vi "TSM SSC Digital Configure Single Level.vi"(0 "Digital TSM In":T2, 5 "Level Type to Set":T1, 7 "Setting":dbl, 11 "error in":errorcluster) -> (4 "Digital TSM Out":T2, 15 "error out":errorcluster)   [LabVIEW 2020]
doc: "Configures and applies the specified single level to the specified pin(s) and pin group(s)."
uses:
  TSM/TSM SSC Digital.ctl
  <vilib>/NI_TestStand_SemiconductorModule/NI_TestStand_Semiconductor_Module.lvlibp/PinMap/Digital Pattern/PinQueryContext/DigitalPatternPinQueryContext.lvclass
  SSC Digital/SSC Digital.ctl
  SSC Digital/Pin Levels and Timing/SSC Digital Single Level Selection.ctl
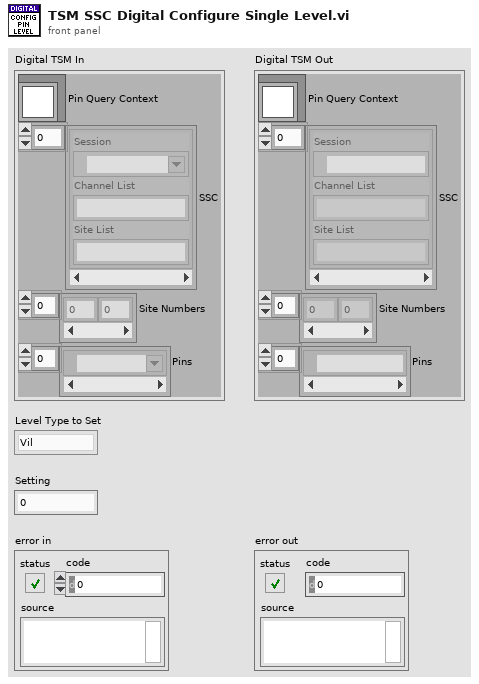
[diagram p1: front panel]
types:
  T1 = typedef "SSC Digital Single Level Selection.ctl" = enum16{"Vil", "Vih", "Vol", "Voh", "Vterm", "Iol", "Ioh", "Vcom"}
  T2 = typedef "TSM SSC Digital.ctl" = cluster{"Pin Query Context":refnum<class "DigitalPatternPinQueryContext.lvclass">, "SSC":T3[], "Site Numbers":i32[], "Pins":tag[]}
  T3 = typedef "SSC Digital.ctl" = cluster{"Session":refnum<k15>, "Channel List":string, "Site List":string}
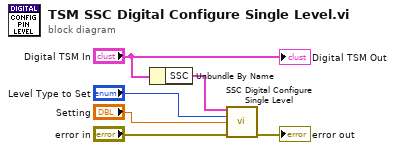
[diagram p0: block diagram]
diagram:
  n1 = Unbundle By Name("Digital TSM In") -> ("SSC"=w5:T3[])
  n2 = call "SSC Digital Configure Single Level.vi"("Digital SSC in"=w5, "Level Type to Set"="Level Type to Set", "Setting"="Setting", "error in"="error in") -> ("error out"=→"error out":errorcluster)  [unwired: 10 in, 1 out]
  "Digital TSM Out" <- "Digital TSM In"
